vi "Decrypt Message.vi"(8 "Error In":errorcluster, 10 "Message":string, 11 "Log in":refnum<class "Log.lvclass">) -> (0 "Error Out":errorcluster, 2 "Decrypted Message":string, 3 "Log out":refnum<class "Log.lvclass">)   [LabVIEW 2019, in "TSC Event Logger.lvlib" / "Log.lvclass"]
uses:
  Log.lvclass
  Encryption/Encryption.lvclass
  Log Sinks/Log Sinks.lvclass
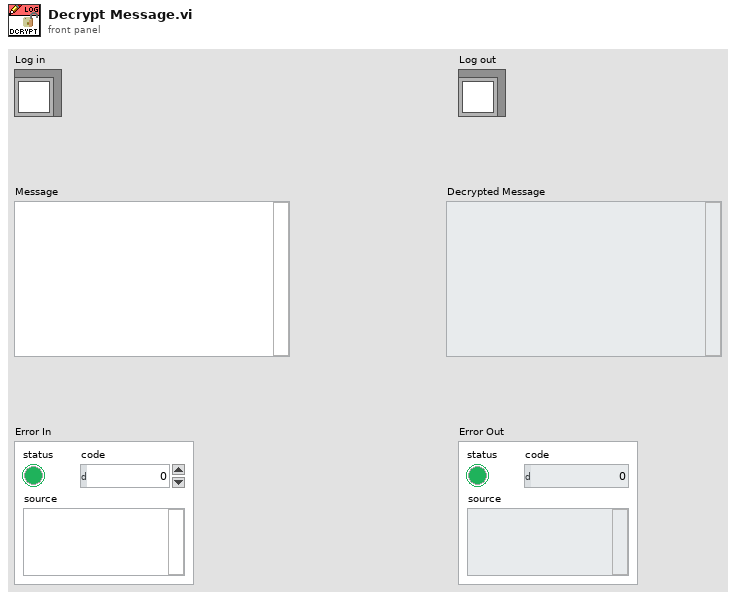
[diagram p1: front panel]
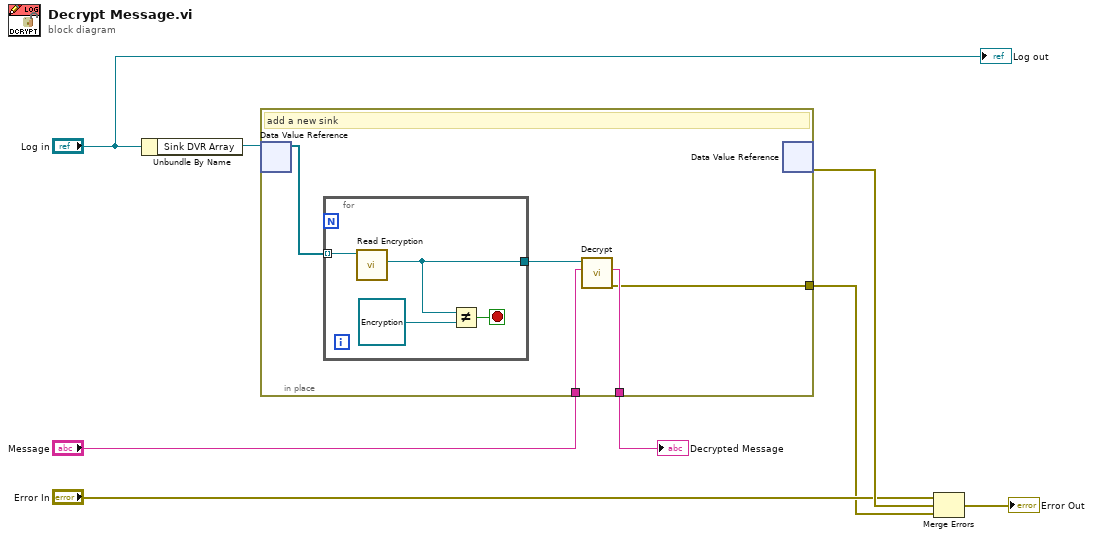
[diagram p0: block diagram]
diagram:
  n1 = Unbundle By Name("Log in") -> ("Sink DVR Array"=w4:refnum<data-value>)
  n2 = in-place {
    in-place-border: "Message" -> [w11]
    in-place-border: [w10] -> w2
    in-place-border: [w9] -> w1
    # "add a new sink"
    n3 = in-place-dvr #1(w4) -> (w13:refnum<class "Log Sinks.lvclass">[])  [unwired: 1 out]
    n4 = for {
      tunnel: w13 -> [w17] mode=indexing
      tunnel: [w14] -> w12
      stop <- w15 stop-if-true
      n5 = call "Read Encryption.vi"("Log Sinks in"=w17) -> ("Encryption"=w14:refnum<class "Encryption.lvclass">)  [unwired: 8 in, 2 out]
      n6 = Not Equal?(x=w14, y=refnum<class "Encryption.lvclass"> refnum ("TSC Event Logger.lvlib:Encryption.lvclass")) -> (x != y?=w15:bool)
    }
    n7 = call-dynamic "Decrypt.vi"("Message"=w11, "Encryption in"=w12) -> ("error out"=w9:errorcluster, "Decrypted Message"=w10:string)  [unwired: 7 in, 1 out]
    n8 = in-place-dvr #1() -> (w7:errorcluster)  [unwired: 1 in, 1 out]
  }
  "Decrypted Message" <- w2
  n9 = Merge Errors("Error In", w7, w1) -> (→"Error Out":errorcluster)
  "Log out" <- "Log in"
